vi "Test AI.vi"() -> ()   [LabVIEW 2012]
uses:
  <vilib>/DAQmx/read.llb/DAQmx Read (Analog 2D DBL NChan NSamp).vi
  <vilib>/DAQmx/create/channels.llb/DAQmx Create Channel (AI-Voltage-Basic).vi
  <vilib>/DAQmx/configure/timing.llb/DAQmx Timing (Sample Clock).vi
  <vilib>/DAQmx/miscellaneous.llb/DAQmx Fill In Error Info.vi
  <resource>/objmgr/daqmx.rc
panel:
  in  "maximum value":dbl=5.0 format="%0.2f"
  out "Waveform Chart":dbl[][](graph)
  in  "stop":bool
  out "data":dbl[][](array[numeric]) format="%0.2f"
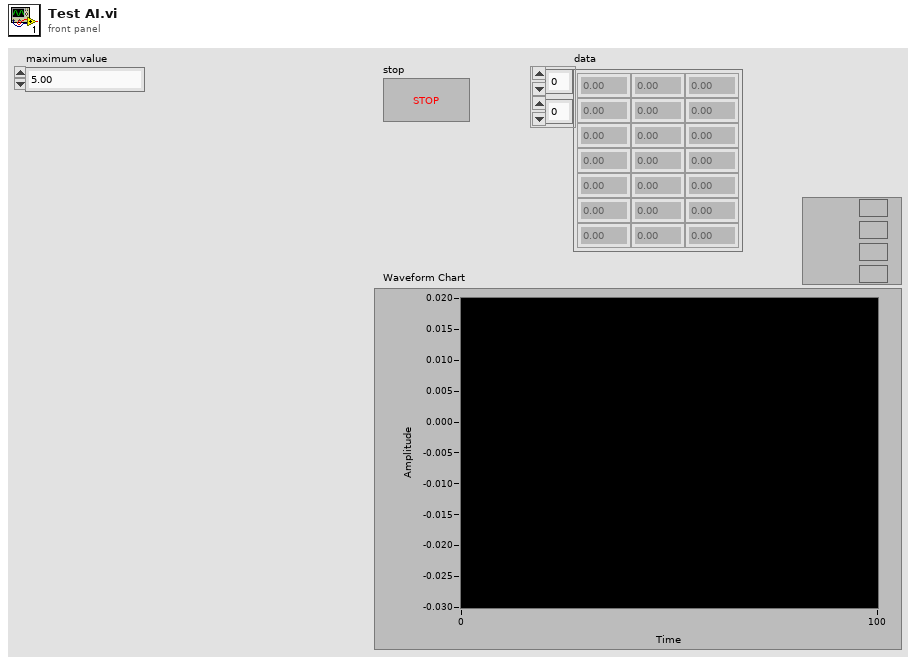
[diagram p1: front panel]
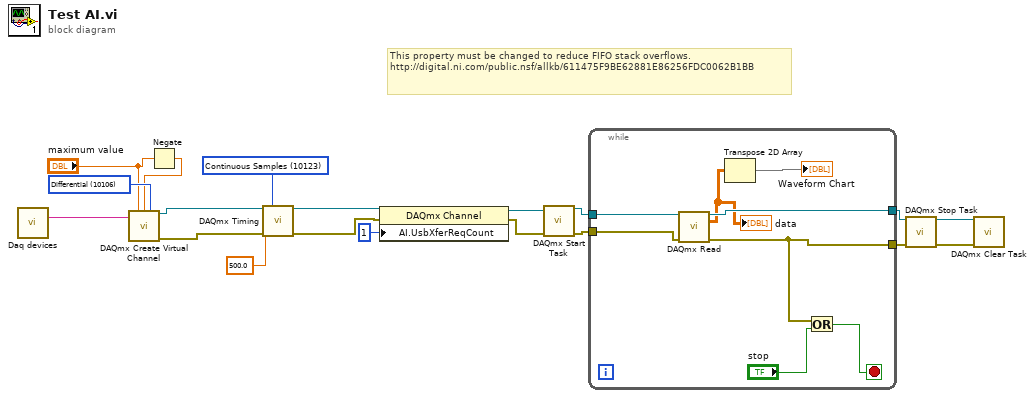
[diagram p0: block diagram]
diagram:
  w10 = 10123 items=["Finite Samples"=10178, "Continuous Samples"=10123, "Hardware Timed Single Point"=12522] ("sample mode")
  w16 = 10106 items=["default"=-1, "RSE"=10083, "NRSE"=10078, "Differential"=10106, "Pseudodifferential"=12529] ("input terminal configuration")
  # "This property must be changed to reduce FIFO stack overflows.\nhttp://digital.ni.com/public.nsf/allkb/611475F9BE62881E86256FDC0062B1BB"
  n1 = call "Daq devices.vi"() -> ("AI"=w1:string)  [unwired: 6 in, 4 out]
  n2 = Negate(x="maximum value") -> (-x=w2:dbl)
  n3 = call-poly <vilib>:"DAQmx Create Virtual Channel.vi"("maximum value"="maximum value", "minimum value"=w2, "input terminal configuration"=w16, "physical channels"=w1) -> ("task out"=w14:refnum<k21>, "error out"=w13:errorcluster)  [unwired: 10 in]
  n4 = call-poly <vilib>:"DAQmx Timing.vi"("task/channels in"=w14, "sample mode"=w10, "rate"=500.0, "error in"=w13) -> ("task out"=w7:refnum<k21>, "error out"=w6:errorcluster)  [unwired: 10 in]
  n5 = property class="DAQmx Channel"(reference=w7, error in=w6, "AI.UsbXferReqCount"=u32 1) -> (reference out=w5:refnum<k21>, error out=w4:errorcluster)
  n6 = call <vilib>:"DAQmx Start Task.vi"("task/channels in"=w5, "error in"=w4) -> ("task out"=w12:refnum<k21>, "error out"=w11:errorcluster)  [unwired: 12 in]
  n7 = while {
    tunnel: [w27] -> w18
    tunnel: [w24] -> w17
    tunnel: w12 -> [w26]
    tunnel: w11 -> [w25]
    stop <- w22 stop-if-true
    n8 = call-poly <vilib>:"DAQmx Read.vi"("task/channels in"=w26, "error in"=w25) -> ("task out"=w27:refnum<k21>, "data"=w21:dbl[][], "error out"=w24:errorcluster)  [unwired: 11 in]
    "data" <- w21
    n9 = Transpose 2D Array(2D array=w21) -> (transposed array=→"Waveform Chart":dbl[][])
    n10 = Or(x=w24, y="stop") -> (x .or. y?=w22:bool)
  }
  n11 = call <vilib>:"DAQmx Stop Task.vi"("task/channels in"=w18, "error in"=w17) -> ("task out"=w9:refnum<k21>, "error out"=w19:errorcluster)  [unwired: 12 in]
  n12 = call <vilib>:"DAQmx Clear Task.vi"("task in"=w9, "error in"=w19) -> ()  [unwired: 13 in, 1 out]
